vi "Get Engine.vi"(8 "error in (no error)":errorcluster, 11 "ts-api in":refnum<class "teststand-api.lvclass">) -> (0 "error out":errorcluster, 3 "ts-api out":refnum<class "teststand-api.lvclass">)   [LabVIEW 2014, in "teststand-api.lvlib" / "teststand-api.lvclass"]
uses:
  teststand-api.lvclass
  teststand-api.lvclass/teststand-api.ctl
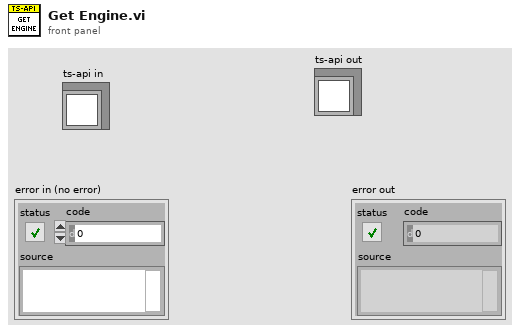
[diagram p1: front panel]
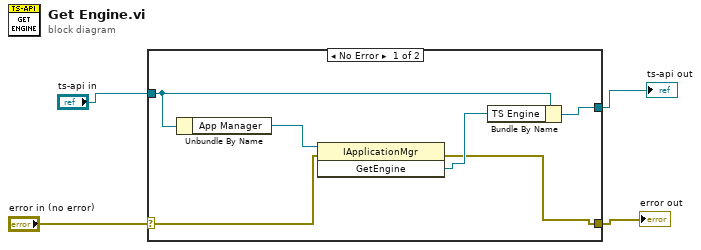
[diagram p0: block diagram]
diagram:
  n1 = case shown="No Error" "error in (no error)" {
    selector: "error in (no error)" -> [w7 w12]
    tunnel: [w5 w12] -> w3
    tunnel: "ts-api in" -> [w10 w11]
    tunnel: [w9 w11] -> w1
    frame No Error {
      n2 = Unbundle By Name(w10) -> ("App Manager"=w8:refnum<k7>)
      n3 = invoke class="IApplicationMgr" method="GetEngine"(reference=w8, error in=w7) -> (error out=w5:errorcluster, "GetEngine"=w6:refnum<k7>)  [unwired: 1 in, 1 out]
      n4 = Bundle By Name(cluster=w10, "TS Engine"=w6) -> (w9:refnum<class "teststand-api.lvclass">)
    }
    frame Error {
    }
  }
  "ts-api out" <- w1
  "error out" <- w3
